vi "AFM_Driver_Manager.StopAllDrivers.vi"(8 "error in (no error)":errorcluster, 11 "AFM_Driver_Manager in":refnum<class "AFM_Driver_Manager.lvclass">) -> (0 "error out":errorcluster, 3 "AFM_Driver_Manager out":refnum<class "AFM_Driver_Manager.lvclass">)   [LabVIEW 2019, in "AFM_Driver_Manager.lvclass"]
uses:
  AFM_Driver_Manager.lvclass
  AFM_Driver_Manager.lvclass/AFM_Driver_Manager.ctl
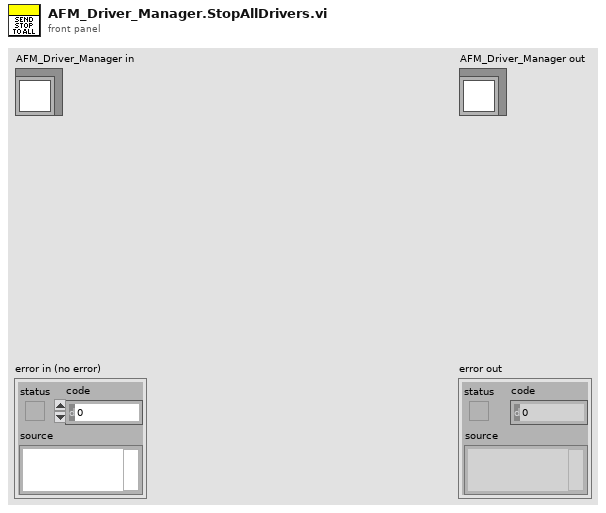
[diagram p1: front panel]
types:
  T1 = typedef "AFM_Driver_Manager.lvclass/AFM_Driver_Manager.PublicMethods.ctl" = cluster{"Stop Event":refnum<user-event>, "Lithography Data":refnum<user-event>, "Run Lithography":refnum<user-event>, "Background Image":refnum<user-event>, "Abort Notifier":refnum<user-event>}
  T2 = cluster{"VI Refnum":refnum<vi>, "Path":path, "Name":string, "Events":T1}[]
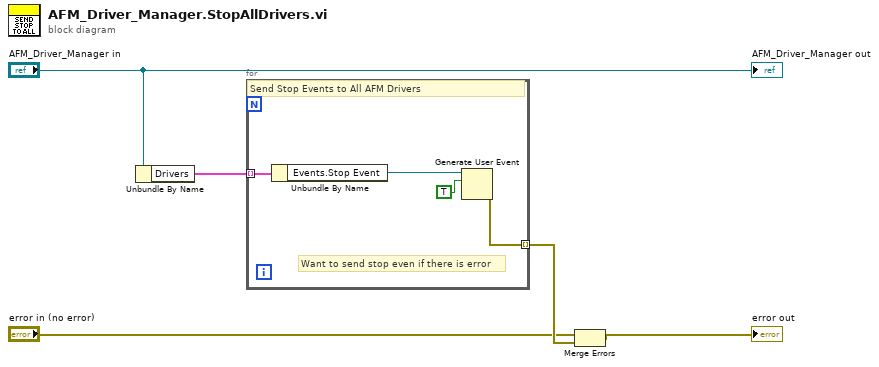
[diagram p0: block diagram]
diagram:
  n1 = Unbundle By Name("AFM_Driver_Manager in") -> ("Drivers"=w5:T2)
  n2 = for {
    tunnel: w5 -> [w8] mode=indexing
    tunnel: [w7] -> w3 mode=indexing
    # "Want to send stop even if there is error"
    # "Send Stop Events to All AFM Drivers"
    n3 = Unbundle By Name(w8) -> ("Events.Stop Event"=w9:refnum<user-event>)
    n4 = Generate User Event(user event=w9, event data cluster=TRUE ("event data")) -> (error out=w7:errorcluster)  [unwired: 2 in, 1 out]
  }
  n5 = Merge Errors("error in (no error)", w3) -> (→"error out":errorcluster)
  "AFM_Driver_Manager out" <- "AFM_Driver_Manager in"
